vi "FuzzyEx Car Backward Parking.vi"() -> ()   [LabVIEW 2023]
doc: "This example demonstrates how you can use fuzzy logic to park a vehicle in a specified location."
uses:
  <vilib>/addons/Fuzzy Logic/TypeDefs/FL System.ctl
  <vilib>/addons/Fuzzy Logic/TypeDefs/FL Variable.ctl
  <vilib>/addons/Fuzzy Logic/TypeDefs/FL Membership Function.ctl
  <vilib>/addons/Fuzzy Logic/TypeDefs/FL Membership Function Shape.ctl
  <vilib>/addons/Fuzzy Logic/TypeDefs/FL Rule.ctl
  <vilib>/addons/Fuzzy Logic/TypeDefs/FL Antecedent.ctl
  <vilib>/addons/Fuzzy Logic/TypeDefs/FL Modifier.ctl
  <vilib>/addons/Fuzzy Logic/TypeDefs/FL Antecedent Connective.ctl
  <vilib>/addons/Fuzzy Logic/TypeDefs/FL Consequent.ctl
  <vilib>/addons/Fuzzy Logic/TypeDefs/FL Consequent Implication.ctl
  <vilib>/addons/Fuzzy Logic/TypeDefs/FL Defuzzification.ctl
  <vilib>/addons/Fuzzy Logic/TypeDefs/FL Interpolating polynomials.ctl
  <vilib>/addons/Fuzzy Logic/FL Fuzzy Controller (MISO).vi
  <vilib>/addons/Fuzzy Logic/NI_Fuzzy_Logic_API.lvlib
panel:
  out "fuzzy system backward":T1={"input variables"=[{"name"="vehicle-position", "range"=[0.0, 10.0, 0.0, 10.0], "MFs"=[{"name"="left", "shape"=1, "points"=[0.0, 0.0, 1.0, 4.0], "color"=16711680, "user-defined shape index"=0}, {"name"="left-center", "shape"=0, "points"=[3.0, 4.0, 5.0], "color"=3342438, "user-defined shape index"=0}, {"name"="center", "shape"=0, "points"=[4.5, 5.0, 5.5], "color"=255, "user-defined shape index"=0}, {"name"="right-center", "shape"=0, "points"=[5.0, 6.0, 7.0], "color"=16724991, "user-defined shape index"=0}, {"name"="right", "shape"=1, "points"=[6.0, 9.0, 10.0, 10.0], "color"=26214, "user-defined shape index"=0}]}, {"name"="vehicle-orientation", "range"=[-90.0, 270.0, -90.0, 270.0], "MFs"=[{"name"="left-down", "shape"=1, "points"=[-90.0, -90.0, -45.0, 20.000000000000014], "color"=16711680, "user-defined shape index"=0}, {"name"="left", "shape"=0, "points"=[-20.000000000000014, 20.000000000000014, 70.0], "color"=3342438, "user-defined shape index"=0}, {"name"="left-up", "shape"=0, "points"=[45.0, 70.0, 90.0], "color"=16724991, "user-defined shape index"=0}, {"name"="up", "shape"=0, "points"=[75.0, 90.0, 104.99999999999999], "color"=255, "user-defined shape index"=0}, {"name"="right-up", "shape"=0, "points"=[90.0, 110.0, 135.0], "color"=10040064, "user-defined shape index"=0}, {"name"="right", "shape"=0, "points"=[110.0, 160.0, 200.0], "color"=13056, "user-defined shape index"=0}, {"name"="right-down", "shape"=1, "points"=[160.0, 225.0, 270.0, 270.0], "color"=26214, "user-defined shape index"=0}]}], "output variables"=[{"name"="steering-angle", "range"=[-30.0, 30.0, -30.0, 30.0], "MFs"=[{"name"="NegBig", "shape"=0, "points"=[-30.0, -30.0, -15.0], "color"=16711680, "user-defined shape index"=0}, {"name"="NegMed", "shape"=0, "points"=[-30.0, -15.0, -4.999999999999999], "color"=3342438, "user-defined shape index"=0}, {"name"="NegSmall", "shape"=0, "points"=[-15.0, -4.999999999999999, 0.0], "color"=16724991, "user-defined shape index"=0}, {"name"="Zero", "shape"=0, "points"=[-4.999999999999999, 0.0, 5.000000000000002], "color"=255, "user-defined shape index"=0}, {"name"="PosSmall", "shape"=0, "points"=[0.0, 5.000000000000002, 15.0], "color"=10040064, "user-defined shape index"=0}, {"name"="PosMed", "shape"=0, "points"=[5.000000000000002, 15.0, 30.0], "color"=13056, "user-defined shape index"=0}, {"name"="PosBig", "shape"=0, "points"=[15.0, 30.0, 30.0], "color"=26214, "user-defined shape index"=0}]}], "rules"=[{"antecedents"=[{"Var Index"=0, "MF Index"=0, "Cond"=0}, {"Var Index"=1, "MF Index"=0, "Cond"=0}], "antecedent connective"=0, "consequents"=[{"Var Index"=0, "MF Index"=2, "Cond"=0}], "consequent implication"=0, "degree of support"=1.0}, {"antecedents"=[{"Var Index"=0, "MF Index"=0, "Cond"=0}, {"Var Index"=1, "MF Index"=1, "Cond"=0}], "antecedent connective"=0, "consequents"=[{"Var Index"=0, "MF Index"=4, "Cond"=0}], "consequent implication"=0, "degree of support"=1.0}, {"antecedents"=[{"Var Index"=0, "MF Index"=0, "Cond"=0}, {"Var Index"=1, "MF Index"=2, "Cond"=0}], "antecedent connective"=0, "consequents"=[{"Var Index"=0, "MF Index"=5, "Cond"=0}], "consequent implication"=0, "degree of support"=1.0}, {"antecedents"=[{"Var Index"=0, "MF Index"=0, "Cond"=0}, {"Var Index"=1, "MF Index"=3, "Cond"=0}], "antecedent connective"=0, "consequents"=[{"Var Index"=0, "MF Index"=5, "Cond"=0}], "consequent implication"=0, "degree of support"=1.0}, {"antecedents"=[{"Var Index"=0, "MF Index"=0, "Cond"=0}, {"Var Index"=1, "MF Index"=4, "Cond"=0}], "antecedent connective"=0, "consequents"=[{"Var Index"=0, "MF Index"=6, "Cond"=0}], "consequent implication"=0, "degree of support"=1.0}, {"antecedents"=[{"Var Index"=0, "MF Index"=0, "Cond"=0}, {"Var Index"=1, "MF Index"=5, "Cond"=0}], "antecedent connective"=0, "consequents"=[{"Var Index"=0, "MF Index"=6, "Cond"=0}], "consequent implication"=0, "degree of support"=1.0}, {"antecedents"=[{"Var Index"=0, "MF Index"=0, "Cond"=0}, {"Var Index"=1, "MF Index"=6, "Cond"=0}], "antecedent connective"=0, "consequents"=[{"Var Index"=0, "MF Index"=6, "Cond"=0}], "consequent implication"=0, "degree of support"=1.0}, {"antecedents"=[{"Var Index"=0, "MF Index"=1, "Cond"=0}, {"Var Index"=1, "MF Index"=0, "Cond"=0}], "antecedent connective"=0, "consequents"=[{"Var Index"=0, "MF Index"=1, "Cond"=0}], "consequent implication"=0, "degree of support"=1.0}, {"antecedents"=[{"Var Index"=0, "MF Index"=1, "Cond"=0}, {"Var Index"=1, "MF Index"=1, "Cond"=0}], "antecedent connective"=0, "consequents"=[{"Var Index"=0, "MF Index"=2, "Cond"=0}], "consequent implication"=0, "degree of support"=1.0}, {"antecedents"=[{"Var Index"=0, "MF Index"=1, "Cond"=0}, {"Var Index"=1, "MF Index"=2, "Cond"=0}], "antecedent connective"=0, "consequents"=[{"Var Index"=0, "MF Index"=4, "Cond"=0}], "consequent implication"=0, "degree of support"=1.0}, {"antecedents"=[{"Var Index"=0, "MF Index"=1, "Cond"=0}, {"Var Index"=1, "MF Index"=3, "Cond"=0}], "antecedent connective"=0, "consequents"=[{"Var Index"=0, "MF Index"=5, "Cond"=0}], "consequent implication"=0, "degree of support"=1.0}, {"antecedents"=[{"Var Index"=0, "MF Index"=1, "Cond"=0}, {"Var Index"=1, "MF Index"=4, "Cond"=0}], "antecedent connective"=0, "consequents"=[{"Var Index"=0, "MF Index"=5, "Cond"=0}], "consequent implication"=0, "degree of support"=1.0}, {"antecedents"=[{"Var Index"=0, "MF Index"=1, "Cond"=0}, {"Var Index"=1, "MF Index"=5, "Cond"=0}], "antecedent connective"=0, "consequents"=[{"Var Index"=0, "MF Index"=6, "Cond"=0}], "consequent implication"=0, "degree of support"=1.0}, {"antecedents"=[{"Var Index"=0, "MF Index"=1, "Cond"=0}, {"Var Index"=1, "MF Index"=6, "Cond"=0}], "antecedent connective"=0, "consequents"=[{"Var Index"=0, "MF Index"=6, "Cond"=0}], "consequent implication"=0, "degree of support"=1.0}, {"antecedents"=[{"Var Index"=0, "MF Index"=2, "Cond"=0}, {"Var Index"=1, "MF Index"=0, "Cond"=0}], "antecedent connective"=0, "consequents"=[{"Var Index"=0, "MF Index"=1, "Cond"=0}], "consequent implication"=0, "degree of support"=1.0}, {"antecedents"=[{"Var Index"=0, "MF Index"=2, "Cond"=0}, {"Var Index"=1, "MF Index"=1, "Cond"=0}], "antecedent connective"=0, "consequents"=[{"Var Index"=0, "MF Index"=1, "Cond"=0}], "consequent implication"=0, "degree of support"=1.0}, {"antecedents"=[{"Var Index"=0, "MF Index"=2, "Cond"=0}, {"Var Index"=1, "MF Index"=2, "Cond"=0}], "antecedent connective"=0, "consequents"=[{"Var Index"=0, "MF Index"=2, "Cond"=0}], "consequent implication"=0, "degree of support"=1.0}, {"antecedents"=[{"Var Index"=0, "MF Index"=2, "Cond"=0}, {"Var Index"=1, "MF Index"=3, "Cond"=0}], "antecedent connective"=0, "consequents"=[{"Var Index"=0, "MF Index"=3, "Cond"=0}], "consequent implication"=0, "degree of support"=1.0}, {"antecedents"=[{"Var Index"=0, "MF Index"=2, "Cond"=0}, {"Var Index"=1, "MF Index"=4, "Cond"=0}], "antecedent connective"=0, "consequents"=[{"Var Index"=0, "MF Index"=4, "Cond"=0}], "consequent implication"=0, "degree of support"=1.0}, {"antecedents"=[{"Var Index"=0, "MF Index"=2, "Cond"=0}, {"Var Index"=1, "MF Index"=5, "Cond"=0}], "antecedent connective"=0, "consequents"=[{"Var Index"=0, "MF Index"=5, "Cond"=0}], "consequent implication"=0, "degree of support"=1.0}, {"antecedents"=[{"Var Index"=0, "MF Index"=2, "Cond"=0}, {"Var Index"=1, "MF Index"=6, "Cond"=0}], "antecedent connective"=0, "consequents"=[{"Var Index"=0, "MF Index"=5, "Cond"=0}], "consequent implication"=0, "degree of support"=1.0}, {"antecedents"=[{"Var Index"=0, "MF Index"=3, "Cond"=0}, {"Var Index"=1, "MF Index"=0, "Cond"=0}], "antecedent connective"=0, "consequents"=[{"Var Index"=0, "MF Index"=0, "Cond"=0}], "consequent implication"=0, "degree of support"=1.0}, {"antecedents"=[{"Var Index"=0, "MF Index"=3, "Cond"=0}, {"Var Index"=1, "MF Index"=1, "Cond"=0}], "antecedent connective"=0, "consequents"=[{"Var Index"=0, "MF Index"=0, "Cond"=0}], "consequent implication"=0, "degree of support"=1.0}, {"antecedents"=[{"Var Index"=0, "MF Index"=3, "Cond"=0}, {"Var Index"=1, "MF Index"=2, "Cond"=0}], "antecedent connective"=0, "consequents"=[{"Var Index"=0, "MF Index"=0, "Cond"=0}], "consequent implication"=0, "degree of support"=1.0}, {"antecedents"=[{"Var Index"=0, "MF Index"=3, "Cond"=0}, {"Var Index"=1, "MF Index"=3, "Cond"=0}], "antecedent connective"=0, "consequents"=[{"Var Index"=0, "MF Index"=1, "Cond"=0}], "consequent implication"=0, "degree of support"=1.0}, {"antecedents"=[{"Var Index"=0, "MF Index"=3, "Cond"=0}, {"Var Index"=1, "MF Index"=4, "Cond"=0}], "antecedent connective"=0, "consequents"=[{"Var Index"=0, "MF Index"=1, "Cond"=0}], "consequent implication"=0, "degree of support"=1.0}, {"antecedents"=[{"Var Index"=0, "MF Index"=3, "Cond"=0}, {"Var Index"=1, "MF Index"=5, "Cond"=0}], "antecedent connective"=0, "consequents"=[{"Var Index"=0, "MF Index"=2, "Cond"=0}], "consequent implication"=0, "degree of support"=1.0}, {"antecedents"=[{"Var Index"=0, "MF Index"=3, "Cond"=0}, {"Var Index"=1, "MF Index"=6, "Cond"=0}], "antecedent connective"=0, "consequents"=[{"Var Index"=0, "MF Index"=2, "Cond"=0}], "consequent implication"=0, "degree of support"=1.0}, {"antecedents"=[{"Var Index"=0, "MF Index"=4, "Cond"=0}, {"Var Index"=1, "MF Index"=0, "Cond"=0}], "antecedent connective"=0, "consequents"=[{"Var Index"=0, "MF Index"=0, "Cond"=0}], "consequent implication"=0, "degree of support"=1.0}, {"antecedents"=[{"Var Index"=0, "MF Index"=4, "Cond"=0}, {"Var Index"=1, "MF Index"=1, "Cond"=0}], "antecedent connective"=0, "consequents"=[{"Var Index"=0, "MF Index"=0, "Cond"=0}], "consequent implication"=0, "degree of support"=1.0}, {"antecedents"=[{"Var Index"=0, "MF Index"=4, "Cond"=0}, {"Var Index"=1, "MF Index"=2, "Cond"=0}], "antecedent connective"=0, "consequents"=[{"Var Index"=0, "MF Index"=0, "Cond"=0}], "consequent implication"=0, "degree of support"=1.0}, {"antecedents"=[{"Var Index"=0, "MF Index"=4, "Cond"=0}, {"Var Index"=1, "MF Index"=3, "Cond"=0}], "antecedent connective"=0, "consequents"=[{"Var Index"=0, "MF Index"=1, "Cond"=0}], "consequent implication"=0, "degree of support"=1.0}, {"antecedents"=[{"Var Index"=0, "MF Index"=4, "Cond"=0}, {"Var Index"=1, "MF Index"=4, "Cond"=0}], "antecedent connective"=0, "consequents"=[{"Var Index"=0, "MF Index"=1, "Cond"=0}], "consequent implication"=0, "degree of support"=1.0}, {"antecedents"=[{"Var Index"=0, "MF Index"=4, "Cond"=0}, {"Var Index"=1, "MF Index"=5, "Cond"=0}], "antecedent connective"=0, "consequents"=[{"Var Index"=0, "MF Index"=2, "Cond"=0}], "consequent implication"=0, "degree of support"=1.0}, {"antecedents"=[{"Var Index"=0, "MF Index"=4, "Cond"=0}, {"Var Index"=1, "MF Index"=6, "Cond"=0}], "antecedent connective"=0, "consequents"=[{"Var Index"=0, "MF Index"=2, "Cond"=0}], "consequent implication"=0, "degree of support"=1.0}], "defuzzification method"=0, "description"="Dual input Fuzzy Controller that is used to automate the maneuvering process leading a truck from an arbitrary start position in backward direction to a loading ramp. The Truck is supposed to be run at constant low speed. \n\nThe maneuvering algorithm is represented by an appropriate rule base (knowledge basis).  \n\nThe current maneuvering situation is at least represented by the two linguistic input variables \"vehicle-position\" towards the loading ramp position and \"vehicle-orientation\".\n\nThe controller output variable \"steering-angle\" serves as process command variable. \n\nThis Fuzzy Controller is responsible for the normal backward manneuvering operations.", "user MF interpolating polynomials"=[]} {"user MF interpolating polynomials"."coa_x(y) coeff" format="%.4g"; "user MF interpolating polynomials"."Area(y) coeff" format="%.4g"; "user MF interpolating polynomials"."X(y) coeff" format="%.4g"; "user MF interpolating polynomials"."Y(x) coeff" format="%.4g"; "user MF interpolating polynomials"."Y" format="%.4g"; "user MF interpolating polynomials"."X" format="%.4g"; "defuzzification method" items=["Center of Area", "Modified Center of Area", "Center of Sums", "Center of Maximum", "Mean of Maximum"]; "rules"."consequents"."Var Index" min=0; "rules"."consequents"."Cond" items=["=", "!="]; "rules"."consequents"."MF Index" min=0; "rules"."antecedents"."Var Index" min=0; "rules"."antecedents"."Cond" items=["=", "!="]; "rules"."antecedents"."MF Index" min=0; "rules"."consequent implication" items=["Minimum", "Product"]; "rules"."antecedent connective" items=["AND (Minimum)", "AND (Product)", "OR (Maximum)", "OR (Probabilistic)"]; "output variables"."MFs"."shape" items=["Triangle", "Trapezoid", "Singleton", "Sigmoid", "Gaussian", "User-Defined"]; "input variables"."MFs"."shape" items=["Triangle", "Trapezoid", "Singleton", "Sigmoid", "Gaussian", "User-Defined"]}
  out "fuzzy system forward":T1={"input variables"=[{"name"="vehicle-position", "range"=[0.0, 10.0, 0.0, 10.0], "MFs"=[{"name"="left", "shape"=1, "points"=[0.0, 0.0, 1.0, 4.0], "color"=16711680, "user-defined shape index"=0}, {"name"="left-center", "shape"=0, "points"=[3.0, 4.0, 5.0], "color"=3342438, "user-defined shape index"=0}, {"name"="center", "shape"=0, "points"=[4.5, 5.0, 5.5], "color"=255, "user-defined shape index"=0}, {"name"="right-center", "shape"=0, "points"=[5.0, 6.0, 7.0], "color"=16724991, "user-defined shape index"=0}, {"name"="right", "shape"=1, "points"=[6.0, 9.0, 10.0, 10.0], "color"=26214, "user-defined shape index"=0}]}, {"name"="vehicle-orientation", "range"=[-90.0, 270.0, -90.0, 270.0], "MFs"=[{"name"="left-down", "shape"=1, "points"=[-90.0, -90.0, -45.0, 20.000000000000014], "color"=16711680, "user-defined shape index"=0}, {"name"="left", "shape"=0, "points"=[-20.000000000000014, 20.000000000000014, 70.0], "color"=3342438, "user-defined shape index"=0}, {"name"="left-up", "shape"=0, "points"=[45.0, 70.0, 90.0], "color"=16724991, "user-defined shape index"=0}, {"name"="up", "shape"=0, "points"=[75.0, 90.0, 104.99999999999999], "color"=255, "user-defined shape index"=0}, {"name"="right-up", "shape"=0, "points"=[90.0, 110.0, 135.0], "color"=10040064, "user-defined shape index"=0}, {"name"="right", "shape"=0, "points"=[110.0, 160.0, 200.0], "color"=13056, "user-defined shape index"=0}, {"name"="right-down", "shape"=1, "points"=[160.0, 225.0, 270.0, 270.0], "color"=26214, "user-defined shape index"=0}]}], "output variables"=[{"name"="steering-angle", "range"=[-30.0, 30.0, -30.0, 30.0], "MFs"=[{"name"="NegBig", "shape"=0, "points"=[-30.0, -30.0, -15.0], "color"=16711680, "user-defined shape index"=0}, {"name"="NegMed", "shape"=0, "points"=[-30.0, -15.0, -4.999999999999999], "color"=3342438, "user-defined shape index"=0}, {"name"="NegSmall", "shape"=0, "points"=[-15.0, -4.999999999999999, 0.0], "color"=16724991, "user-defined shape index"=0}, {"name"="Zero", "shape"=0, "points"=[-4.999999999999999, 0.0, 5.000000000000002], "color"=255, "user-defined shape index"=0}, {"name"="PosSmall", "shape"=0, "points"=[0.0, 5.000000000000002, 15.0], "color"=10040064, "user-defined shape index"=0}, {"name"="PosMed", "shape"=0, "points"=[5.000000000000002, 15.0, 30.0], "color"=13056, "user-defined shape index"=0}, {"name"="PosBig", "shape"=0, "points"=[15.0, 30.0, 30.0], "color"=26214, "user-defined shape index"=0}]}], "rules"=[{"antecedents"=[{"Var Index"=0, "MF Index"=0, "Cond"=0}, {"Var Index"=1, "MF Index"=0, "Cond"=0}], "antecedent connective"=0, "consequents"=[{"Var Index"=0, "MF Index"=6, "Cond"=0}], "consequent implication"=0, "degree of support"=1.0}, {"antecedents"=[{"Var Index"=0, "MF Index"=0, "Cond"=0}, {"Var Index"=1, "MF Index"=1, "Cond"=0}], "antecedent connective"=0, "consequents"=[{"Var Index"=0, "MF Index"=6, "Cond"=0}], "consequent implication"=0, "degree of support"=1.0}, {"antecedents"=[{"Var Index"=0, "MF Index"=0, "Cond"=0}, {"Var Index"=1, "MF Index"=2, "Cond"=0}], "antecedent connective"=0, "consequents"=[{"Var Index"=0, "MF Index"=5, "Cond"=0}], "consequent implication"=0, "degree of support"=1.0}, {"antecedents"=[{"Var Index"=0, "MF Index"=0, "Cond"=0}, {"Var Index"=1, "MF Index"=3, "Cond"=0}], "antecedent connective"=0, "consequents"=[{"Var Index"=0, "MF Index"=5, "Cond"=0}], "consequent implication"=0, "degree of support"=1.0}, {"antecedents"=[{"Var Index"=0, "MF Index"=0, "Cond"=0}, {"Var Index"=1, "MF Index"=4, "Cond"=0}], "antecedent connective"=0, "consequents"=[{"Var Index"=0, "MF Index"=4, "Cond"=0}], "consequent implication"=0, "degree of support"=1.0}, {"antecedents"=[{"Var Index"=0, "MF Index"=0, "Cond"=0}, {"Var Index"=1, "MF Index"=5, "Cond"=0}], "antecedent connective"=0, "consequents"=[{"Var Index"=0, "MF Index"=2, "Cond"=0}], "consequent implication"=0, "degree of support"=1.0}, {"antecedents"=[{"Var Index"=0, "MF Index"=0, "Cond"=0}, {"Var Index"=1, "MF Index"=6, "Cond"=0}], "antecedent connective"=0, "consequents"=[{"Var Index"=0, "MF Index"=0, "Cond"=0}], "consequent implication"=0, "degree of support"=1.0}, {"antecedents"=[{"Var Index"=0, "MF Index"=1, "Cond"=0}, {"Var Index"=1, "MF Index"=0, "Cond"=0}], "antecedent connective"=0, "consequents"=[{"Var Index"=0, "MF Index"=6, "Cond"=0}], "consequent implication"=0, "degree of support"=1.0}, {"antecedents"=[{"Var Index"=0, "MF Index"=1, "Cond"=0}, {"Var Index"=1, "MF Index"=1, "Cond"=0}], "antecedent connective"=0, "consequents"=[{"Var Index"=0, "MF Index"=6, "Cond"=0}], "consequent implication"=0, "degree of support"=1.0}, {"antecedents"=[{"Var Index"=0, "MF Index"=1, "Cond"=0}, {"Var Index"=1, "MF Index"=2, "Cond"=0}], "antecedent connective"=0, "consequents"=[{"Var Index"=0, "MF Index"=5, "Cond"=0}], "consequent implication"=0, "degree of support"=1.0}, {"antecedents"=[{"Var Index"=0, "MF Index"=1, "Cond"=0}, {"Var Index"=1, "MF Index"=3, "Cond"=0}], "antecedent connective"=0, "consequents"=[{"Var Index"=0, "MF Index"=5, "Cond"=0}], "consequent implication"=0, "degree of support"=1.0}, {"antecedents"=[{"Var Index"=0, "MF Index"=1, "Cond"=0}, {"Var Index"=1, "MF Index"=4, "Cond"=0}], "antecedent connective"=0, "consequents"=[{"Var Index"=0, "MF Index"=4, "Cond"=0}], "consequent implication"=0, "degree of support"=1.0}, {"antecedents"=[{"Var Index"=0, "MF Index"=1, "Cond"=0}, {"Var Index"=1, "MF Index"=5, "Cond"=0}], "antecedent connective"=0, "consequents"=[{"Var Index"=0, "MF Index"=2, "Cond"=0}], "consequent implication"=0, "degree of support"=1.0}, {"antecedents"=[{"Var Index"=0, "MF Index"=1, "Cond"=0}, {"Var Index"=1, "MF Index"=6, "Cond"=0}], "antecedent connective"=0, "consequents"=[{"Var Index"=0, "MF Index"=1, "Cond"=0}], "consequent implication"=0, "degree of support"=1.0}, {"antecedents"=[{"Var Index"=0, "MF Index"=2, "Cond"=0}, {"Var Index"=1, "MF Index"=0, "Cond"=0}], "antecedent connective"=0, "consequents"=[{"Var Index"=0, "MF Index"=5, "Cond"=0}], "consequent implication"=0, "degree of support"=1.0}, {"antecedents"=[{"Var Index"=0, "MF Index"=2, "Cond"=0}, {"Var Index"=1, "MF Index"=1, "Cond"=0}], "antecedent connective"=0, "consequents"=[{"Var Index"=0, "MF Index"=5, "Cond"=0}], "consequent implication"=0, "degree of support"=1.0}, {"antecedents"=[{"Var Index"=0, "MF Index"=2, "Cond"=0}, {"Var Index"=1, "MF Index"=2, "Cond"=0}], "antecedent connective"=0, "consequents"=[{"Var Index"=0, "MF Index"=4, "Cond"=0}], "consequent implication"=0, "degree of support"=1.0}, {"antecedents"=[{"Var Index"=0, "MF Index"=2, "Cond"=0}, {"Var Index"=1, "MF Index"=3, "Cond"=0}], "antecedent connective"=0, "consequents"=[{"Var Index"=0, "MF Index"=3, "Cond"=0}], "consequent implication"=0, "degree of support"=1.0}, {"antecedents"=[{"Var Index"=0, "MF Index"=2, "Cond"=0}, {"Var Index"=1, "MF Index"=4, "Cond"=0}], "antecedent connective"=0, "consequents"=[{"Var Index"=0, "MF Index"=2, "Cond"=0}], "consequent implication"=0, "degree of support"=1.0}, {"antecedents"=[{"Var Index"=0, "MF Index"=2, "Cond"=0}, {"Var Index"=1, "MF Index"=5, "Cond"=0}], "antecedent connective"=0, "consequents"=[{"Var Index"=0, "MF Index"=1, "Cond"=0}], "consequent implication"=0, "degree of support"=1.0}, {"antecedents"=[{"Var Index"=0, "MF Index"=2, "Cond"=0}, {"Var Index"=1, "MF Index"=6, "Cond"=0}], "antecedent connective"=0, "consequents"=[{"Var Index"=0, "MF Index"=1, "Cond"=0}], "consequent implication"=0, "degree of support"=1.0}, {"antecedents"=[{"Var Index"=0, "MF Index"=3, "Cond"=0}, {"Var Index"=1, "MF Index"=0, "Cond"=0}], "antecedent connective"=0, "consequents"=[{"Var Index"=0, "MF Index"=5, "Cond"=0}], "consequent implication"=0, "degree of support"=1.0}, {"antecedents"=[{"Var Index"=0, "MF Index"=3, "Cond"=0}, {"Var Index"=1, "MF Index"=1, "Cond"=0}], "antecedent connective"=0, "consequents"=[{"Var Index"=0, "MF Index"=4, "Cond"=0}], "consequent implication"=0, "degree of support"=1.0}, {"antecedents"=[{"Var Index"=0, "MF Index"=3, "Cond"=0}, {"Var Index"=1, "MF Index"=2, "Cond"=0}], "antecedent connective"=0, "consequents"=[{"Var Index"=0, "MF Index"=2, "Cond"=0}], "consequent implication"=0, "degree of support"=1.0}, {"antecedents"=[{"Var Index"=0, "MF Index"=3, "Cond"=0}, {"Var Index"=1, "MF Index"=3, "Cond"=0}], "antecedent connective"=0, "consequents"=[{"Var Index"=0, "MF Index"=1, "Cond"=0}], "consequent implication"=0, "degree of support"=1.0}, {"antecedents"=[{"Var Index"=0, "MF Index"=3, "Cond"=0}, {"Var Index"=1, "MF Index"=4, "Cond"=0}], "antecedent connective"=0, "consequents"=[{"Var Index"=0, "MF Index"=1, "Cond"=0}], "consequent implication"=0, "degree of support"=1.0}, {"antecedents"=[{"Var Index"=0, "MF Index"=3, "Cond"=0}, {"Var Index"=1, "MF Index"=5, "Cond"=0}], "antecedent connective"=0, "consequents"=[{"Var Index"=0, "MF Index"=0, "Cond"=0}], "consequent implication"=0, "degree of support"=1.0}, {"antecedents"=[{"Var Index"=0, "MF Index"=3, "Cond"=0}, {"Var Index"=1, "MF Index"=6, "Cond"=0}], "antecedent connective"=0, "consequents"=[{"Var Index"=0, "MF Index"=0, "Cond"=0}], "consequent implication"=0, "degree of support"=1.0}, {"antecedents"=[{"Var Index"=0, "MF Index"=4, "Cond"=0}, {"Var Index"=1, "MF Index"=0, "Cond"=0}], "antecedent connective"=0, "consequents"=[{"Var Index"=0, "MF Index"=5, "Cond"=0}], "consequent implication"=0, "degree of support"=1.0}, {"antecedents"=[{"Var Index"=0, "MF Index"=4, "Cond"=0}, {"Var Index"=1, "MF Index"=1, "Cond"=0}], "antecedent connective"=0, "consequents"=[{"Var Index"=0, "MF Index"=4, "Cond"=0}], "consequent implication"=0, "degree of support"=1.0}, {"antecedents"=[{"Var Index"=0, "MF Index"=4, "Cond"=0}, {"Var Index"=1, "MF Index"=2, "Cond"=0}], "antecedent connective"=0, "consequents"=[{"Var Index"=0, "MF Index"=2, "Cond"=0}], "consequent implication"=0, "degree of support"=1.0}, {"antecedents"=[{"Var Index"=0, "MF Index"=4, "Cond"=0}, {"Var Index"=1, "MF Index"=3, "Cond"=0}], "antecedent connective"=0, "consequents"=[{"Var Index"=0, "MF Index"=1, "Cond"=0}], "consequent implication"=0, "degree of support"=1.0}, {"antecedents"=[{"Var Index"=0, "MF Index"=4, "Cond"=0}, {"Var Index"=1, "MF Index"=4, "Cond"=0}], "antecedent connective"=0, "consequents"=[{"Var Index"=0, "MF Index"=1, "Cond"=0}], "consequent implication"=0, "degree of support"=1.0}, {"antecedents"=[{"Var Index"=0, "MF Index"=4, "Cond"=0}, {"Var Index"=1, "MF Index"=5, "Cond"=0}], "antecedent connective"=0, "consequents"=[{"Var Index"=0, "MF Index"=0, "Cond"=0}], "consequent implication"=0, "degree of support"=1.0}, {"antecedents"=[{"Var Index"=0, "MF Index"=4, "Cond"=0}, {"Var Index"=1, "MF Index"=6, "Cond"=0}], "antecedent connective"=0, "consequents"=[{"Var Index"=0, "MF Index"=0, "Cond"=0}], "consequent implication"=0, "degree of support"=1.0}], "defuzzification method"=0, "description"="Dual input Fuzzy Controller that is used to automate the maneuvering process leading a truck from an arbitrary start position in backward direction to a loading ramp. The Truck is supposed to be run at constant low speed. \n\nThe maneuvering algorithm is represented by an appropriate rule base (knowledge basis).  \n\nThe current maneuvering situation is at least represented by the two linguistic input variables \"vehicle-position\" towards the loading ramp position and \"vehicle-orientation\".\n\nThe controller output variable \"steering-angle\" serves as process command variable. \n\nThis Fuzzy Controller is responsible for foreward maneuvering operations necessary to bring the vehicle in a good start position when backward operation fails to hit the ramp.. ", "user MF interpolating polynomials"=[]} {"user MF interpolating polynomials"."coa_x(y) coeff" format="%.4g"; "user MF interpolating polynomials"."Area(y) coeff" format="%.4g"; "user MF interpolating polynomials"."X(y) coeff" format="%.4g"; "user MF interpolating polynomials"."Y(x) coeff" format="%.4g"; "user MF interpolating polynomials"."Y" format="%.4g"; "user MF interpolating polynomials"."X" format="%.4g"; "defuzzification method" items=["Center of Area", "Modified Center of Area", "Center of Sums", "Center of Maximum", "Mean of Maximum"]; "rules"."consequents"."Var Index" min=0; "rules"."consequents"."Cond" items=["=", "!="]; "rules"."consequents"."MF Index" min=0; "rules"."antecedents"."Var Index" min=0; "rules"."antecedents"."Cond" items=["=", "!="]; "rules"."antecedents"."MF Index" min=0; "rules"."consequent implication" items=["Minimum", "Product"]; "rules"."antecedent connective" items=["AND (Minimum)", "AND (Product)", "OR (Maximum)", "OR (Probabilistic)"]; "output variables"."MFs"."shape" items=["Triangle", "Trapezoid", "Singleton", "Sigmoid", "Gaussian", "User-Defined"]; "input variables"."MFs"."shape" items=["Triangle", "Trapezoid", "Singleton", "Sigmoid", "Gaussian", "User-Defined"]}
  in  "Activate Fuzzy Controller":bool
  out "Steering Angle":picture
  out "Arrived":bool
  out "Steering Wheel":dbl
  in  "Initial Vehicle Angle":dbl(knob)=-56.0 min=-90.0 max=270.0 step=1.0 scale=-90.0..270.0
  in  "Stop":bool
  out "Grid":cluster{dbl[], dbl[]}[](graph)
  out "Car parking":picture
  # "Overview: Demonstrates the use of fuzzy logic to simulate parking a vehicle in a specified location.\nInstructions:\n1. Run the VI.\n2. Move the cursor to set the vehicle initial position and specify an initial vehicle angle.\n3. Click Activate Fuzzy Controller to park the vehicle using Fuzzy Logic and verify the car moving to the garage.\n4. Click Stop to stop the VI."
  # "Garage"
  # "IF"
  # "THEN"
  # "IF"
  # "THEN"
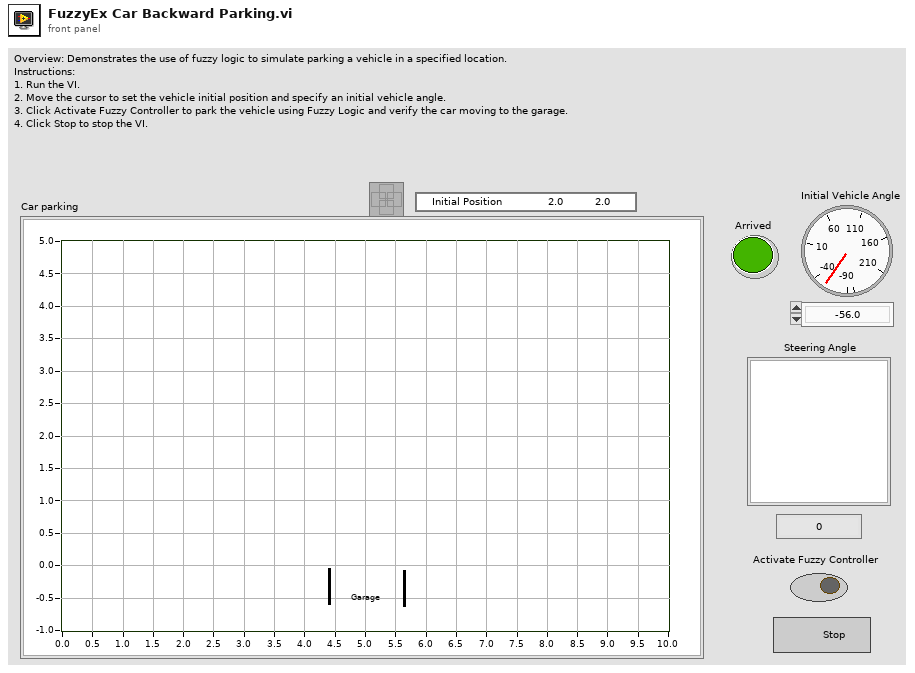
[diagram p1: front panel]
types:
  T1 = typedef "NI_Fuzzy_Logic_API.lvlib/FL System.ctl" = cluster{"input variables":T2[], "output variables":T2[], "rules":T5[], "defuzzification method":T11, "description":string, "user MF interpolating polynomials":T12[]}
  T2 = typedef "NI_Fuzzy_Logic_API.lvlib/FL Variable.ctl" = cluster{"name":string, "range":dbl[], "MFs":T3[]}
  T3 = typedef "NI_Fuzzy_Logic_API.lvlib/FL Membership Function.ctl" = cluster{"name":string, "shape":T4, "points":dbl[], "color":u32, "user-defined shape index":i32}
  T4 = typedef "NI_Fuzzy_Logic_API.lvlib/FL Membership Function Shape.ctl" = u16
  T5 = typedef "NI_Fuzzy_Logic_API.lvlib/FL Rule.ctl" = cluster{"antecedents":T6[], "antecedent connective":T8, "consequents":T9[], "consequent implication":T10, "degree of support":dbl}
  T6 = typedef "NI_Fuzzy_Logic_API.lvlib/FL Antecedent.ctl" = cluster{"Var Index":i32, "MF Index":i32, "Cond":T7}
  T7 = typedef "NI_Fuzzy_Logic_API.lvlib/FL Modifier.ctl" = u16
  T8 = typedef "NI_Fuzzy_Logic_API.lvlib/FL Antecedent Connective.ctl" = u16
  T9 = typedef "NI_Fuzzy_Logic_API.lvlib/FL Consequent.ctl" = cluster{"Var Index":i32, "MF Index":i32, "Cond":T7}
  T10 = typedef "NI_Fuzzy_Logic_API.lvlib/FL Consequent Implication.ctl" = u16
  T11 = typedef "NI_Fuzzy_Logic_API.lvlib/FL Defuzzification.ctl" = u16
  T12 = typedef "NI_Fuzzy_Logic_API.lvlib/FL Interpolating polynomials.ctl" = cluster{"X":dbl[], "Y":dbl[], "Y(x) coeff":dbl[][], "X(y) coeff":dbl[][], "Area(y) coeff":dbl[][], "coa_x(y) coeff":dbl[][]}
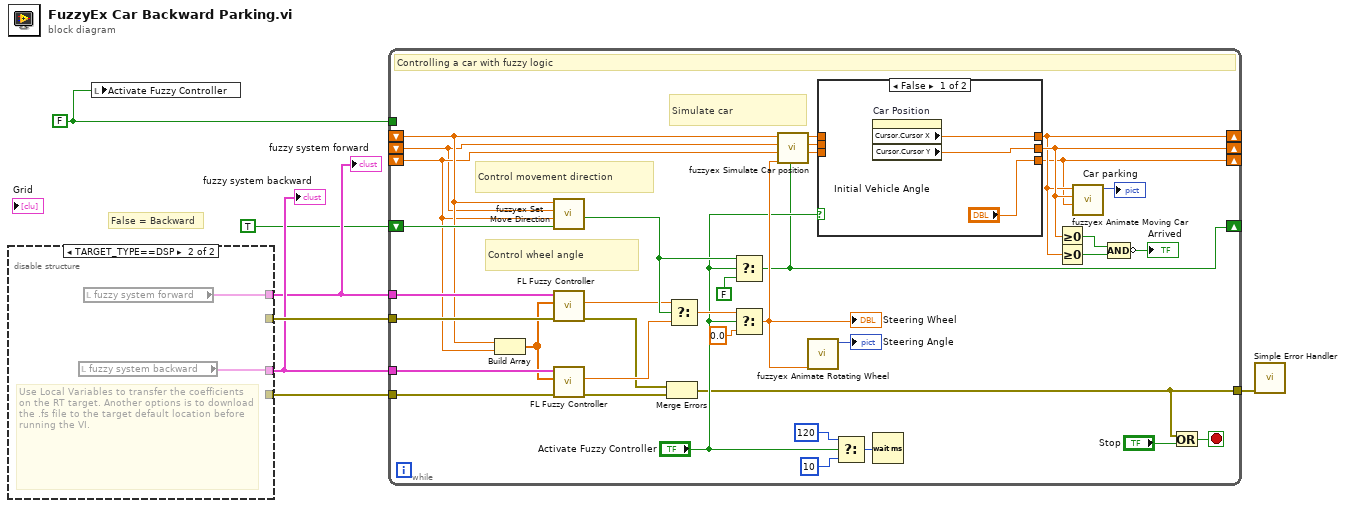
[diagram p0: block diagram]
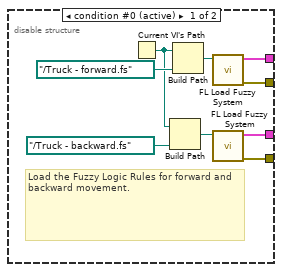
[diagram p2: hidden frame]
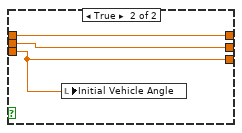
[diagram p3: hidden frame]
diagram:
  w3 = FALSE ("Operation Mode")
  # "False = Backward"
  n1 = disable-structure shown="TARGET_TYPE==DSP" {
    disable-tunnel: [w16 _] -> w7
    disable-tunnel: [w11 _] -> w6
    disable-tunnel: [w10 w17] -> w5
    disable-tunnel: [w9 w18] -> w4
    frame condition #0 (active) {
      # "Load the Fuzzy Logic Rules for forward and backward movement."
      n2 = Current VI's Path() -> (path=w8:path)
      n3 = Build Path(base path=w8, name or relative path=path "../Truck - backward.fs") -> (appended path=w14:path)
      n4 = Build Path(base path=w8, name or relative path=path "../Truck - forward.fs") -> (appended path=w15:path)
      n5 = call <vilib>:"FL Load Fuzzy System.vi"("file path"=w15) -> ("error out"=w16:errorcluster, "fuzzy system out"=w9:T1)  [unwired: 1 in, 8 out]
      n6 = call <vilib>:"FL Load Fuzzy System.vi"("file path"=w14) -> ("error out"=w11:errorcluster, "fuzzy system out"=w10:T1)  [unwired: 1 in, 8 out]
    }
    frame condition #1 {
      # "Use Local Variables to transfer the coefficients on the RT target. Another options is to download the .fs file to the target default location before running the VI."
      n7 = local read "fuzzy system backward"() -> (w17:T1)
      n8 = local read "fuzzy system forward"() -> (w18:T1)
    }
  }
  "fuzzy system forward" <- w4
  "fuzzy system backward" <- w5
  n9 = local write "Activate Fuzzy Controller"(w3) -> ()
  n10 = while {
    tunnel: w7 -> [w48]
    tunnel: w4 -> [w49]
    shift-left: TRUE -> [w52]
    shift-right: [w22] -> _
    shift-left: _ -> [w45]
    shift-right: [w42] -> _
    shift-left: _ -> [w24]
    shift-right: [w39] -> _
    shift-left: _ -> [w23]
    shift-right: [w43] -> _
    tunnel: w3 -> [_]
    tunnel: w5 -> [w44]
    tunnel: w6 -> [w35]
    tunnel: [w28] -> w2
    stop <- w27 stop-if-true
    # "Control wheel angle"
    # "Simulate car"
    # "Control movement direction"
    # "Controlling a car with fuzzy logic"
    n11 = Build Array(w45, w24) -> (w34:dbl[])
    n12 = call "fuzzyex Set Move Direction.vi"("direction"=w52, "beta"=w24, "y(VC)"=w23, "x(VC)"=w45) -> ("New Dir"=w40:bool)
    n13 = call-poly <vilib>:"FL Fuzzy Controller.vi"("error in (no error)"=w48, "input values"=w34, "fuzzy system in"=w49) -> ("error out"=w30:errorcluster, "output value"=w33:dbl)  [unwired: 7 out]
    n14 = call-poly <vilib>:"FL Fuzzy Controller.vi"("error in (no error)"=w35, "input values"=w34, "fuzzy system in"=w44) -> ("error out"=w29:errorcluster, "output value"=w32:dbl)  [unwired: 7 out]
    n15 = Merge Errors(w30, w29) -> (w28:errorcluster)
    n16 = Select(t=w33, s=w40, f=w32) -> (s? t:f=w51:dbl)
    n17 = Select(t=w40, s="Activate Fuzzy Controller", f=FALSE) -> (s? t:f=w22:bool)
    n18 = Select(t=w51, s="Activate Fuzzy Controller", f=0.0) -> (s? t:f=w47:dbl)
    "Steering Wheel" <- w47
    n19 = call "fuzzyex Simulate Car position.vi"("Direction"=w22, "Steering Angle (Phi)"=w47, "Current Vehicle Orientation (Beta)"=w24, "Current Position Y"=w23, "Current Position X"=w45) -> ("New Vehicle Orientation Beta"=w36:dbl, "New position Y"=w37:dbl, "New position X"=w38:dbl)  [unwired: 2 out]
    n20 = call "fuzzyex Animate Rotating Wheel.vi"("Angle (deg)"=w47) -> ("new picture"=→"Steering Angle":picture)  [unwired: 10 out]
    n21 = case shown="False" "Activate Fuzzy Controller" {
      tunnel: w37 -> [_ w60]
      tunnel: w38 -> [_ w61]
      tunnel: w36 -> [_ w59]
      tunnel: [w56 w60] -> w43
      tunnel: [w58 w61] -> w42
      tunnel: ["Initial Vehicle Angle" w59] -> w39
      frame False {
        n22 = property on="Car Position" class="XYGraph (strict)"() -> ("Cursor.Cursor X"=w58:dbl, "Cursor.Cursor Y"=w56:dbl)  [unwired: 2 in, 2 out]
      }
      frame True {
        n23 = local write "Initial Vehicle Angle"(w59) -> ()
      }
    }
    n24 = Select(t=u32 120, s="Activate Fuzzy Controller", f=u32 10) -> (s? t:f=w55:u32)
    n25 = Wait (ms)(milliseconds to wait=w55) -> ()  [unwired: 1 out]
    n26 = Greater Or Equal To 0?(x=w43) -> (x >= 0?=w54:bool)
    n27 = Greater Or Equal To 0?(x=w42) -> (x >= 0?=w53:bool)
    n28 = call "fuzzyex Animate Moving Car.vi"("Car Angle (deg)"=w39, "y position"=w43, "x position"=w42) -> ("new picture"=→"Car parking":picture)  [unwired: 8 out]
    n29 = Compound Arithmetic op=AND(w54, w53) -> (invert →"Arrived":bool)
    n30 = Or(x=w28, y="Stop") -> (x .or. y?=w27:bool)
  }
  n31 = call <vilib>:"Simple Error Handler.vi"("error in (no error)"=w2) -> ()  [unwired: 4 in, 5 out]
